vi "Initialize.vi"(11 "2 Lines?":bool) -> ()   [LabVIEW 2019, in "HD44780.lvlib"]
uses:
  HD44780.lvlib
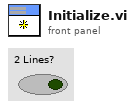
[diagram p1: front panel]
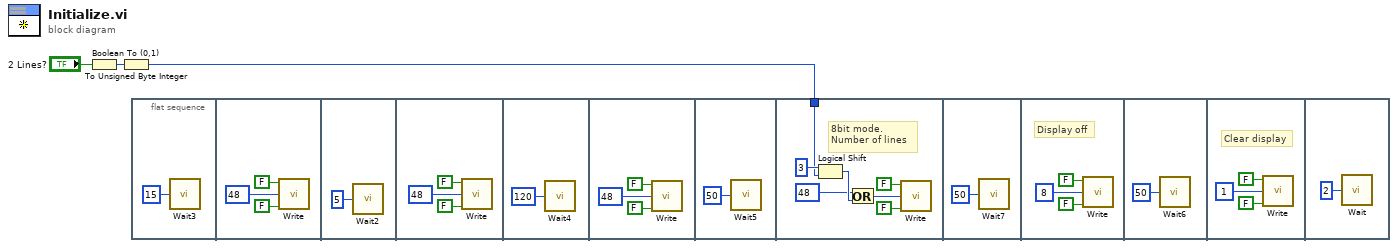
[diagram p0: block diagram]
diagram:
  n1 = Boolean To (0,1)(Boolean="2 Lines?") -> (0, 1=w2:i16)
  n2 = To Unsigned Byte Integer(number=w2) -> (unsigned 8bit integer=w1:u8)
  n3 = flat-sequence {
    tunnel: w1 -> [w21]
    frame #0 {
      n4 = call "Wait3"("Count(mSec)"=u8 15) -> ()  [unwired: 1 out]
    }
    frame #1 {
      n5 = call "Write.vi"("Check Busy Flag?"=FALSE, "Data"=u8 48, "Register Select"=FALSE) -> ()  [unwired: 9 in]
    }
    frame #2 {
      n6 = call "Wait2"("Count(mSec)"=u8 5) -> ()  [unwired: 1 out]
    }
    frame #3 {
      n7 = call "Write.vi"("Check Busy Flag?"=FALSE, "Data"=u8 48, "Register Select"=FALSE) -> ()  [unwired: 9 in]
    }
    frame #4 {
      n8 = call "Wait4"("Count(uSec)"=u8 120 ("Count(mSec)")) -> ()  [unwired: 1 out]
    }
    frame #5 {
      n9 = call "Write.vi"("Check Busy Flag?"=FALSE, "Data"=u8 48, "Register Select"=FALSE) -> ()  [unwired: 9 in]
    }
    frame #6 {
      n10 = call "Wait5"("Count(uSec)"=u8 50 ("Count(mSec)")) -> ()  [unwired: 1 out]
    }
    frame #7 {
      # "8bit mode.\nNumber of lines"
      n11 = Logical Shift(y=i16 3, x=w21) -> (x << y=w20:u8)
      n12 = Or(x=u8 48 ("Data"), y=w20) -> (x .or. y?=w18:u8)
      n13 = call "Write.vi"("Check Busy Flag?"=FALSE, "Data"=w18, "Register Select"=FALSE) -> ()  [unwired: 9 in]
    }
    frame #8 {
      n14 = call "Wait7"("Count(uSec)"=u8 50 ("Count(mSec)")) -> ()  [unwired: 1 out]
    }
    frame #9 {
      # "Display off"
      n15 = call "Write.vi"("Check Busy Flag?"=FALSE, "Data"=u8 8, "Register Select"=FALSE) -> ()  [unwired: 9 in]
    }
    frame #10 {
      n16 = call "Wait6"("Count(uSec)"=u8 50 ("Count(mSec)")) -> ()  [unwired: 1 out]
    }
    frame #11 {
      # "Clear display"
      n17 = call "Write.vi"("Check Busy Flag?"=FALSE, "Data"=u8 1, "Register Select"=FALSE) -> ()  [unwired: 9 in]
    }
    frame #12 {
      n18 = call "Wait"("Count(mSec)"=u8 2) -> ()  [unwired: 1 out]
    }
  }
